vi "cs_usb_read.vi"(5 "handle":i32) -> (0 "Error":bool, 2 "string":string)   [LabVIEW 2017]
uses:
  kernel32.dll
panel:
  out "size 2":i32
  out "output":i8[](array[numeric])
  in  "btc_byteArray":u8[](array[numeric])
  in  "bufOutput 64 bytes":u8[](array[numeric])=[0, 0, 0, 0, 0, 0, 0, 0, 0, 0, 0, 0, 0, 0, 0, 0, 0, 0, 0, 0, 0, 0, 0, 0, 0, 0, 0, 0, 0, 0, 0, 0, 0, 0, 0, 0, 0, 0, 0, 0, 0, 0, 0, 0, 0, 0, 0, 0, 0, 0, 0, 0, 0, 0, 0, 0, 0, 0, 0, 0, 0, 0, 0, 0] format="%x"
  in  "BULK_TRANSFER_CONTROL":cluster{"Numeric":u32}={"Numeric"=2}
  in  "overlapp":i32
  in  "size":i32
  out "outp-size":i32=2
  in  "outp":i32
  out "btcsize":i32=2
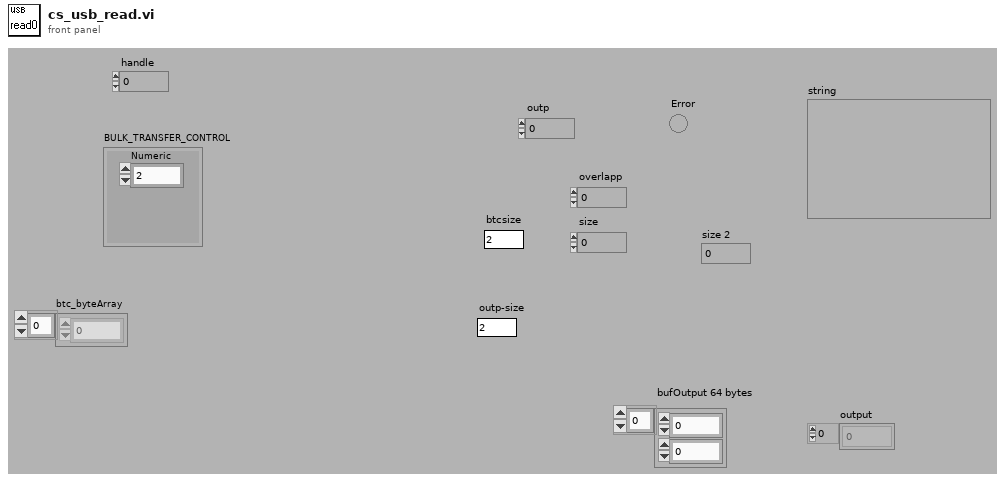
[diagram p1: front panel]
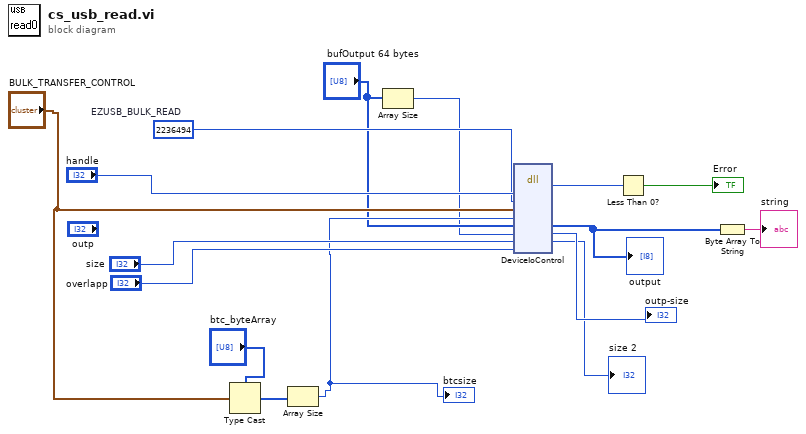
[diagram p0: block diagram]
diagram:
  w11 = u32 2236494  # EZUSB_BULK_READ
  n1 = Type Cast(type="btc_byteArray", x="BULK_TRANSFER_CONTROL") -> (*(type *) &x=w9:u8[])
  n2 = Array Size(array=w9) -> (size(s)=w7:i32)
  "btcsize" <- w7
  n3 = Array Size(array="bufOutput 64 bytes") -> (size(s)=w4:i32)
  n4 = dll-call lib="kernel32.dll" fn="DeviceIoControl" label="DeviceIOControl"("handle"="handle", "vier-const"=w11, "BULK_TRANSFER_CONTROL"="BULK_TRANSFER_CONTROL", "inputsize"=w7, "output"="bufOutput 64 bytes", "outputsize"=w4, "size"="size", "overlapp"="overlapp") -> ("ltemp"=w12:i32, "output"=w2:i8[], "outputsize"=→"outp-size":i32, "size"=→"size 2":i32)  [unwired: 8 in, 2 out]
  "output" <- w2
  n5 = Less Than 0?(x=w12) -> (x < 0?=→"Error":bool)
  n6 = Byte Array To String(unsigned byte array=w2) -> (string=→"string":string)
